vi "Initialize Keithley DMM.vi"(8 "error in (no error)":errorcluster, 10 "Serial Configuration":T1={"Baud Rate (19200)"=19200, "Flow Control (1: XON/XOFF)"=1, "Termination Char (0:CR)"=0} {"Termination Char (0:CR)" items=["CR", "LF"]; "Flow Control (1: XON/XOFF)" items=["None", "XON/XOFF", "RTS/CTS (2701 Only)", "XON/XOFF & RTS/CTS (2701 Only)"]; "Baud Rate (19200)" items=["300"=300, "600"=600, "1200"=1200, "2400"=2400, "4800"=4800, "9600"=9600, "19.2k"=19200, "38.4k (2701 Only)"=38400, "57.6k (2701 Only)"=57600, "115.2k (2701 Only)"=115200]}, 11 "VISA resource name":refnum<visa-resource-name>) -> (0 "error out":errorcluster, 3 "VISA resource name out":refnum<visa-resource-name>)   [LabVIEW 2015]
uses:
  <instrlib>/Keithley 27XX/Keithley 27XX.lvlib
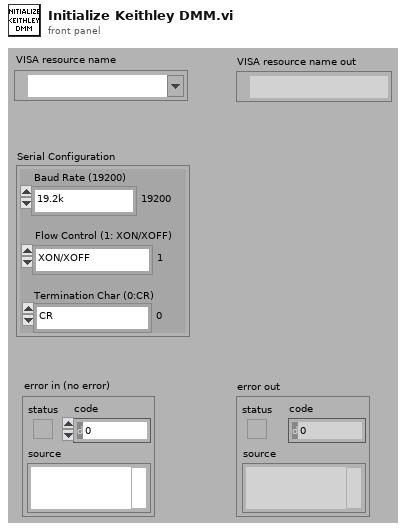
[diagram p1: front panel]
types:
  T1 = cluster{"Baud Rate (19200)":u32, "Flow Control (1: XON/XOFF)":u16, "Termination Char (0:CR)":u16}
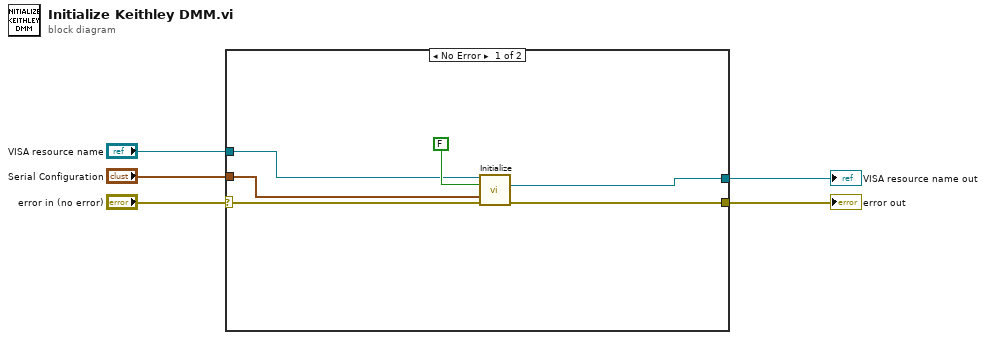
[diagram p0: block diagram]
diagram:
  n1 = case shown="No Error" "error in (no error)" {
    selector: "error in (no error)" -> [w9 w12]
    tunnel: [w10 w12] -> w5
    tunnel: "VISA resource name" -> [w7 _]
    tunnel: "Serial Configuration" -> [w8 _]
    tunnel: [w6 _] -> w1
    frame No Error {
      n2 = call <instrlib>:"Initialize.vi"("VISA resource name"=w7, "ID Query? (T: Yes)"=FALSE, "Serial Configuration"=w8, "error in (no error)"=w9) -> ("VISA resource name out"=w6:refnum<visa-resource-name>, "error out"=w10:errorcluster)  [unwired: 10 in]
    }
    frame Error {
    }
  }
  "error out" <- w5
  "VISA resource name out" <- w1
